vi "Index.vi"(8 "error in (no error)":errorcluster, 10 "Index":i32, 11 "U32 Array in":refnum<class "U32 Array.lvclass">) -> (0 "error out":errorcluster, 3 "Indexed element":refnum<class "Generic Data.lvclass">)   [LabVIEW 2020, in "Data.lvlib" / "U32 Array.lvclass"]
doc: "Index an element from 'Generic Data in'.\nThis implementation returns a generic U32 class with the indexed U32."
uses:
  U32 Array.lvclass
  Generic Data.lvclass
  U32 Array.lvclass/U32 Array.ctl
  U32/U32.lvclass/U32.ctl
  U32/U32.lvclass
  C:/Users/Henri/OneDrive/LabVIEW/Framework/Data/Generic Data/Generic Data.lvclass
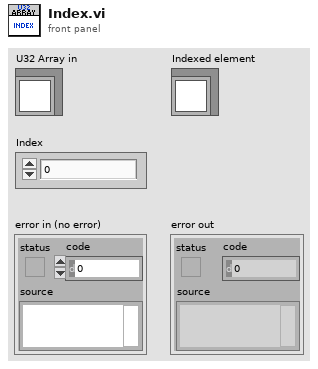
[diagram p1: front panel]
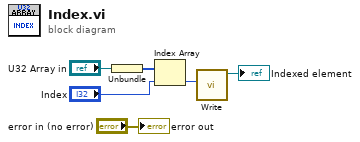
[diagram p0: block diagram]
diagram:
  n1 = Unbundle("U32 Array in") -> (w5:u32[])
  n2 = Index Array(array=w5, index="Index") -> (element=w2:u32)
  n3 = call "Write.vi"("U32"=w2) -> ("U32 out"=→"Indexed element":refnum<class "U32.lvclass">)  [unwired: 10 in]
  "error out" <- "error in (no error)"
